vi "Close SHVs.vi"(8 "error in (no error)":errorcluster, 11 "Cylinder in":refnum<class "Cylinder.lvclass">) -> (0 "error out":errorcluster, 3 "Cylinder out":refnum<class "Cylinder.lvclass">)   [LabVIEW 2015, in "cRIO-Carbondioxide.lvlib" / "CO2-Actor.lvlib" / "Cylinder.lvclass"]
uses:
  Cylinder.lvclass
  Cylinder.lvclass/Cylinder.ctl
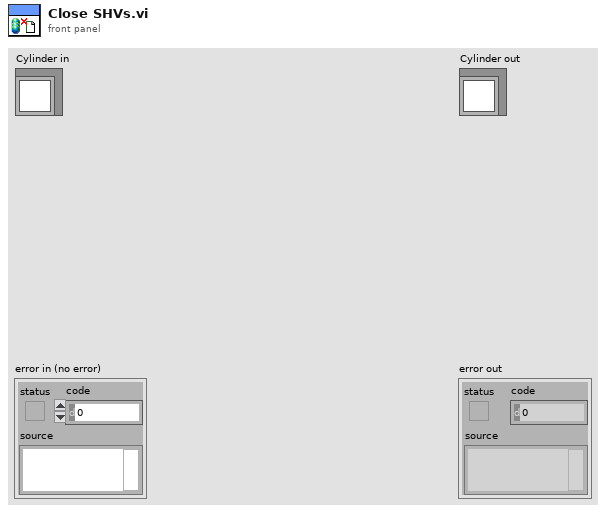
[diagram p1: front panel]
types:
  T1 = cluster{"Pressure Setpoint Control ":refnum<k21>, "Analog output":refnum<k21>, "Direction Valve IO":refnum<k21>, "Home Control":refnum<k21>, "Position Sensor":refnum<k21>}
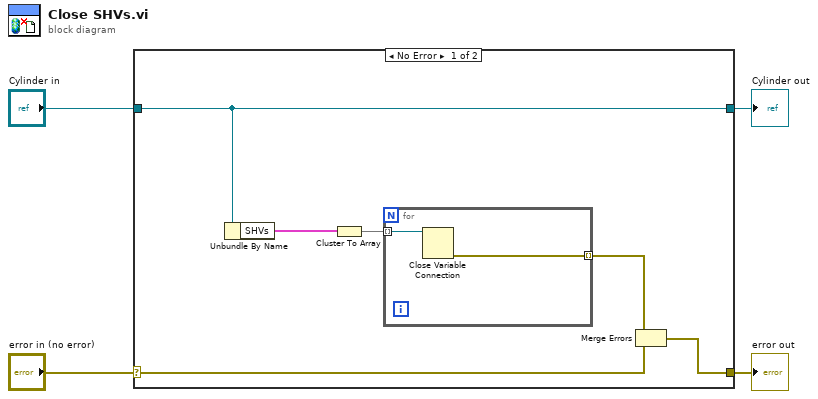
[diagram p0: block diagram]
diagram:
  n1 = case shown="No Error" "error in (no error)" {
    selector: "error in (no error)" -> [w5 w14]
    tunnel: [w6 w14] -> w3
    tunnel: [w9 w13] -> w1
    tunnel: "Cylinder in" -> [w9 w13]
    frame No Error {
      n2 = Unbundle By Name(w9) -> ("SHVs"=w8:T1)
      n3 = Cluster To Array(cluster=w8) -> (array=w10:refnum<k21>[])
      n4 = for {
        tunnel: w10 -> [w12] mode=indexing
        tunnel: [w11] -> w7 mode=indexing
        n5 = Close Variable Connection(11:w12) -> (0:w11:errorcluster)  [unwired: 1 in]
      }
      n6 = Merge Errors(w7, w5) -> (w6:errorcluster)
    }
    frame Error {
    }
  }
  "error out" <- w3
  "Cylinder out" <- w1
